vi "Initialize Hardware.vi"(8 "error in (no error)":errorcluster, 9 "Initialize Parameter":T1={"Ref"=variant, "topology name"="Configured Topology"}, 10 "DAQ Type":enum16{"Hardware", "Simulation"}(ring), 11 "PXIe 2737 in":refnum<class "PXIe 2737.lvclass">) -> (0 "error out":errorcluster, 3 "PXIe 2737 out":refnum<class "PXIe 2737.lvclass">)   [LabVIEW 2021, in "S-Matrix.lvlib" / "PXIe 2737.lvclass"]
uses:
  PXIe 2737.lvclass
  Initialize Parameter.ctl
  S-Matrix.lvlib
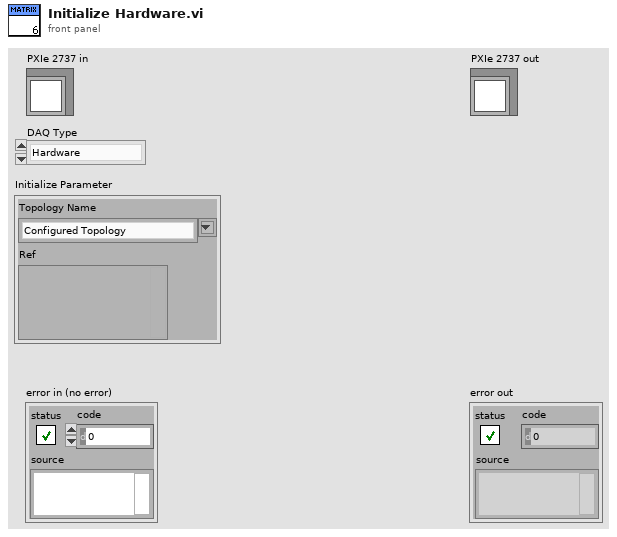
[diagram p1: front panel]
types:
  T1 = typedef "S-Matrix.lvlib/Initialize Parameter.ctl" = cluster{"Ref":variant, "topology name":string}
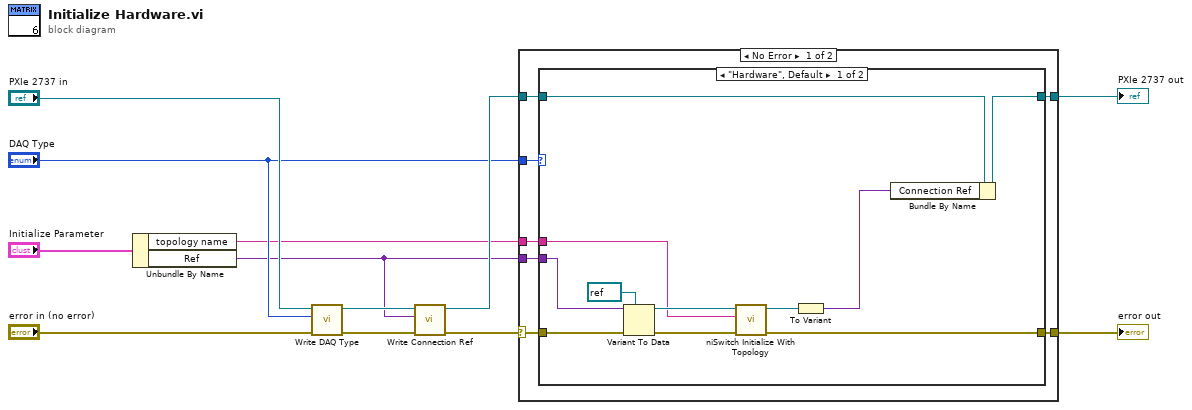
[diagram p0: block diagram]
diagram:
  n1 = Unbundle By Name("Initialize Parameter") -> ("topology name"=w1:string, "Ref"=w2:variant)
  n2 = call-dynamic "Write DAQ Type.vi"("error in (no error)"="error in (no error)", "DAQ Type"="DAQ Type", "PXIe 2737 in"="PXIe 2737 in") -> ("error out"=w11:errorcluster, "PXIe 2737 out"=w8:refnum<class "PXIe 2737.lvclass">)  [unwired: 7 in]
  n3 = call-dynamic "Write Connection Ref.vi"("error in (no error)"=w11, "Connection Ref"=w2, "PXIe 2737 in"=w8) -> ("error out"=w9:errorcluster, "PXIe 2737 out"=w7:refnum<class "PXIe 2737.lvclass">)  [unwired: 7 in]
  n4 = case shown="No Error" w9 {
    selector: w9 -> [w17 w33]
    tunnel: w7 -> [w18 w34]
    tunnel: "DAQ Type" -> [w19 _]
    tunnel: w2 -> [w16 _]
    tunnel: [w15 w34] -> w5
    tunnel: [w14 w33] -> w4
    tunnel: w1 -> [w13 _]
    frame No Error {
      n5 = case shown="\"Hardware\", Default" w19 {
        tunnel: w18 -> [w25 w32]
        tunnel: w17 -> [w30 w31]
        tunnel: w16 -> [w28 _]
        tunnel: [w23 w32] -> w15
        tunnel: [w24 w31] -> w14
        tunnel: w13 -> [w21 _]
        frame "Hardware", Default {
          n6 = Variant To Data(error in=w30, type=refnum<k15> refnum ("resource name"), Variant=w28) -> (data=w27:refnum<k15>, error out=w26:errorcluster)
          n7 = call <instrlib>:"niSwitch Initialize With Topology.vi"("error in (no error)"=w26, "topology name"=w21, "resource name"=w27) -> ("error out"=w24:errorcluster, "instrument handle out"=w22:refnum<k15>)  [unwired: 2 in, 5 out]
          n8 = To Variant(anything=w22) -> (Variant=w20:variant)
          n9 = Bundle By Name(cluster=w25, "Connection Ref"=w20) -> (w23:refnum<class "PXIe 2737.lvclass">)
        }
        frame "Simulation" {
        }
      }
    }
    frame Error {
    }
  }
  "error out" <- w4
  "PXIe 2737 out" <- w5
